vi "ParseGlassData.vi"(11 "Result Set":string[](array[string])) -> (1 "String":string, 2 "Numeric":dbl, 3 "Numeric 2":dbl)   [LabVIEW 2013]
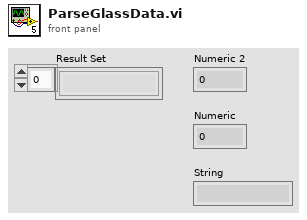
[diagram p1: front panel]
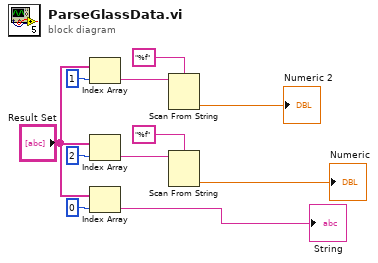
[diagram p0: block diagram]
diagram:
  n1 = Index Array(array="Result Set", index=1) -> (element=w6:string)
  n2 = Index Array(array="Result Set", index=2) -> (element=w11:string)
  n3 = Index Array(array="Result Set", index=0) -> (element=→"String":string)
  n4 = Scan From String(format string="%f", input string=w6) -> (output 1=→"Numeric 2":dbl)  [unwired: 3 in, 3 out]
  n5 = Scan From String(format string="%f", input string=w11) -> (output 1=→"Numeric":dbl)  [unwired: 3 in, 3 out]
